vi "Calibration Helper.vi"(6 "Std Devs":cluster{"H":dbl, "S":dbl, "V":dbl}={"H"=4.0, "S"=6.0, "V"=4.0}, 7 "Image Name":string="untitled", 8 "Color Mode":u16(ring)=2 items=["RGB", "HSL", "HSV", "HSI", "CIE L*a*b*", "CIE XYZ"], 9 "Color Components":T1={"Hue"={110.0, 142.0}, "Sat"={138.0, 255.0}, "Val"={139.0, 198.0}} {"Val" scale=0.0..255.0; "Sat" scale=0.0..255.0; "Hue" scale=0.0..255.0 scale format="%#_3g"}, 10 "Image":T2, 11 "Image Ctl Refnum":refnum<vi>) -> (2 "Changed":bool, 3 "output color":T3)   [LabVIEW 2013]
uses:
  <vilib>/vision/Image Controls.llb/IMAQ Image.ctl
  <vilib>/vision/NI_Vision_Development_Module.lvlib
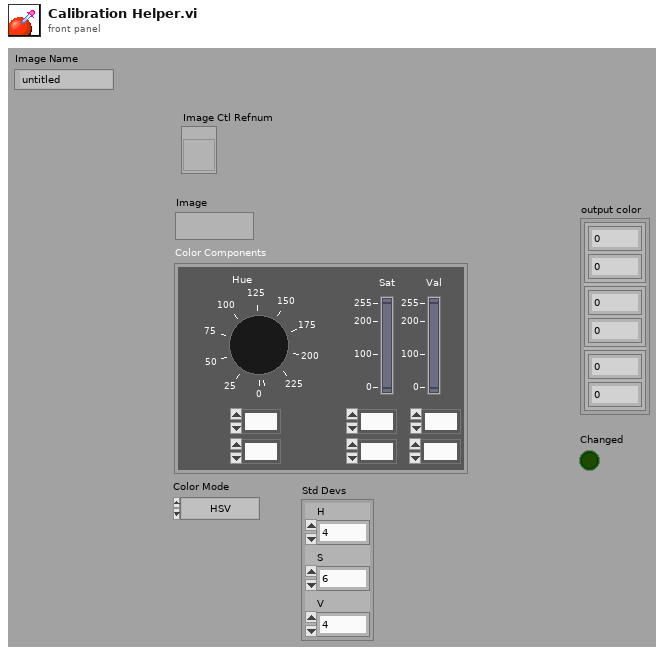
[diagram p1: front panel]
types:
  T1 = cluster{"Hue":cluster{dbl, dbl}, "Sat":cluster{dbl, dbl}, "Val":cluster{dbl, dbl}}
  T2 = typedef "IMAQ Image.ctl" = refnum<image>
  T3 = cluster{cluster{dbl, dbl}, cluster{dbl, dbl}, cluster{dbl, dbl}}
  T4 = typedef "Image Type" = u32
  T5 = cluster{"Global Rectangle":i32[], "Contours":cluster{"Contour Type":u32, "ROI Type":u32, "Points":i32[]}[]}
  T6 = cluster{"histogram":u32[], "Minimal Value":sgl, "Maximal Value":sgl, "Starting Value":sgl, "Interval Width":sgl, "Mean Value":sgl, "Standard  Variation":sgl, "Area (pixels)":i32}
  T7 = cluster{"histogram":u32[], "Minimal Value":sgl, "Maximal Value":sgl, "Starting Value":sgl, "Interval Width":sgl, "Mean Value":sgl, "Standard  Variation":sgl, "Area (pixels)":i32}[]
  T8 = cluster{"[0]":cluster{dbl, dbl}, "[1]":cluster{dbl, dbl}, "[2]":cluster{dbl, dbl}}
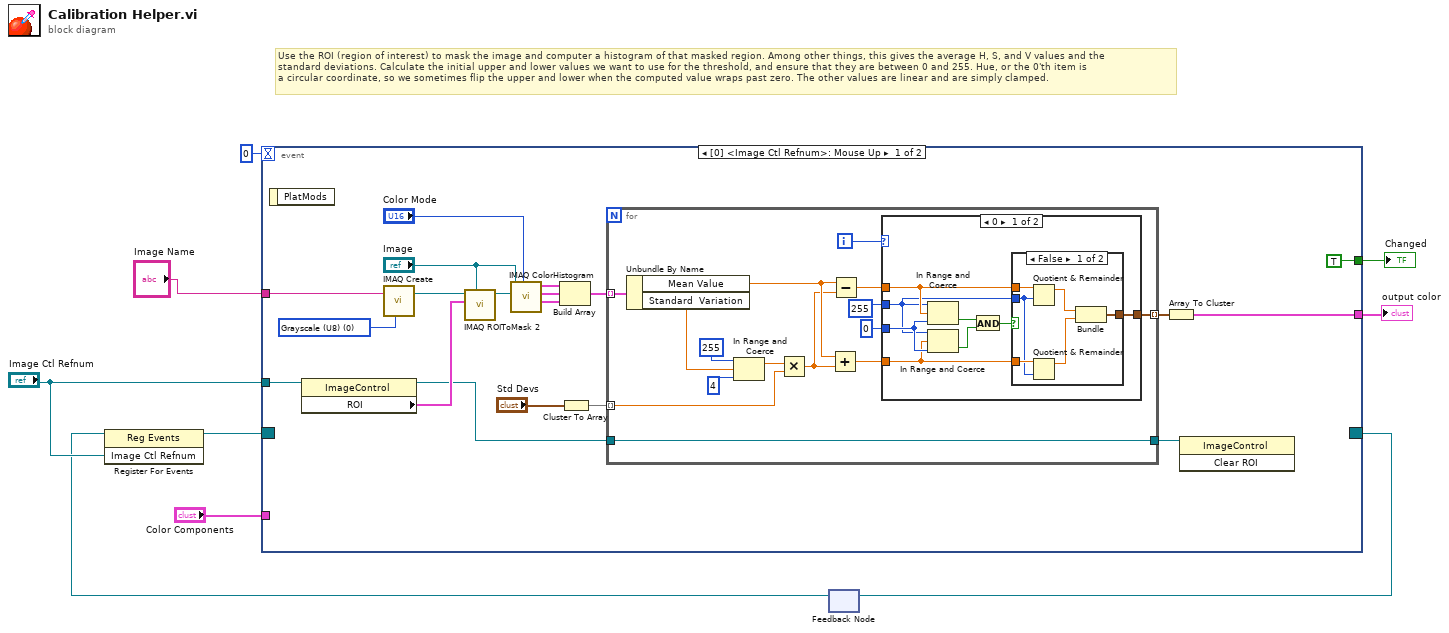
[diagram p0: block diagram]
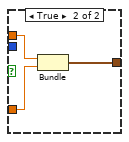
[diagram p2: hidden frame]
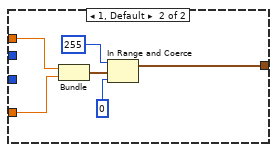
[diagram p3: hidden frame]
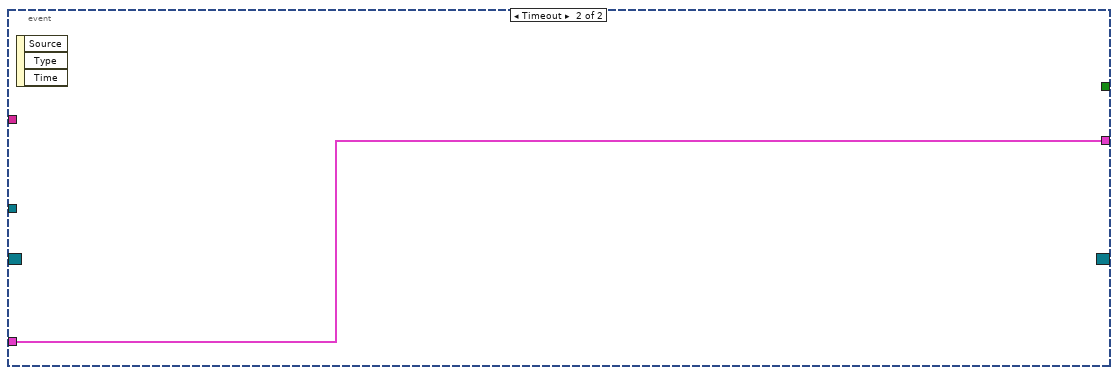
[diagram p4: hidden frame]
diagram:
  # "Use the ROI (region of interest) to mask the image and computer a histogram of that masked region. Among other things, this gives the average H, S, and V values and the\nstandard deviations. Calculate the initial upper and lower values we want to use for the threshold, and ensure that they are between 0 and 255. Hue, or the 0'th item is\na circular coordinate, so we sometimes flip the upper and lower when the computed value wraps past zero. The other values are linear and are simply clamped."
  n1 = feedback #1() -> (w3:refnum<event-registration>)  [unwired: 1 in]
  n2 = register-events(reference=w3, "Image Ctl Refnum") -> (reference out=w7:refnum<event-registration>)  [unwired: 1 in, 1 out]
  n3 = event shown="[0] <Image Ctl Refnum>: Mouse Up" {
    selector: w7 -> [_ _]
    dyn-events: [_ _] -> w4
    timeout: 0 -> [_ _]
    tunnel: "Image Ctl Refnum" -> [w16 _]
    tunnel: "Color Components" -> [_ w67]
    tunnel: [w12 w67] -> w5
    tunnel: [TRUE _] -> w2
    tunnel: "Image Name" -> [w10 _]
    event Mouse Up {
      w28 = T4 0 items=["Grayscale (U8)", "Grayscale (I16)", "Grayscale (SGL)", "Complex (CSG)", "RGB (U32)", "HSL (U32)", "RGB (U64)", "Grayscale (U16)"] ("Image Type")
      n4 = event-data() -> ()  [unwired: 1 in, 1 out]
      n5 = property on="Property Node" class="ImageControl"(reference=w16) -> (reference out=w13:refnum<vi>, "ROI"=w15:T5)  [unwired: 1 in, 1 out]
      n6 = call "IMAQ Create"("Image Name"=w10, "Image Type"=w28) -> ("New Image"=w26:T2)  [unwired: 3 in, 1 out]
      n7 = call "IMAQ ROIToMask 2"("Image Model"="Image", "ROI Descriptor"=w15, "Image"=w26) -> ("Image Out"=w27:T2)  [unwired: 6 in, 2 out]
      n8 = call "IMAQ ColorHistogram"("Color Mode"="Color Mode", "Image Src"="Image", "Image Mask"=w27) -> ("Red or Hue or X or L* Histogram Report"=w22:T6, "Green or Sat or Y or a* Histogram Report"=w21:T6, "Blue or Luma or Val or Inten or Z or b* Histogram Report"=w20:T6)  [unwired: 3 in, 1 out]
      n9 = Build Array(w22, w21, w20) -> (w18:T7)
      n10 = Cluster To Array(cluster="Std Devs") -> (array=w19:dbl[])
      n11 = for {
        tunnel: w19 -> [w39] mode=indexing
        tunnel: w18 -> [w43] mode=indexing
        tunnel: [w34] -> w17 mode=indexing
        tunnel: [w29] -> w14
        tunnel: w13 -> [w29]
        i -> [w32]
        n12 = Unbundle By Name(w43) -> ("Mean Value"=w37:sgl, "Standard  Variation"=w40:sgl)
        n13 = In Range and Coerce(upper limit=255, x=w40, lower limit=4) -> (coerced(x)=w38:sgl)  [unwired: 1 out]
        n14 = Multiply(x=w38, y=w39) -> (x*y=w33:dbl)
        n15 = Add(x=w37, y=w33) -> (x+y=w35:dbl)
        n16 = Subtract(x=w37, y=w33) -> (x-y=w36:dbl)
        n17 = case shown="0" w32 {
          tunnel: w36 -> [w46 w63]
          tunnel: w35 -> [w45 w62]
          tunnel: [w48 w61] -> w34
          tunnel: 255 -> [w44 _]
          tunnel: 0 -> [w47 _]
          frame 0 {
            n18 = In Range and Coerce(upper limit=w44, x=w46, lower limit=w47) -> (In Range?=w50:bool)  [unwired: 1 out]
            n19 = In Range and Coerce(upper limit=w44, x=w45, lower limit=w47) -> (In Range?=w49:bool)  [unwired: 1 out]
            n20 = And(x=w50, y=w49) -> (x .and. y?=w51:bool)
            n21 = case shown="False" w51 {
              tunnel: [w54 w60] -> w48
              tunnel: w46 -> [w57 w58]
              tunnel: w45 -> [w56 w59]
              tunnel: w44 -> [w55 _]
              frame False {
                n22 = Quotient & Remainder(x=w57, y=w55) -> (x-y*floor(x/y)=w52:dbl)  [unwired: 1 out]
                n23 = Quotient & Remainder(x=w56, y=w55) -> (x-y*floor(x/y)=w53:dbl)  [unwired: 1 out]
                n24 = Bundle(w52, w53) -> (w54:cluster{dbl, dbl})  [unwired: 1 in]
              }
              frame True {
                n25 = Bundle(w58, w59) -> (w60:cluster{dbl, dbl})  [unwired: 1 in]
              }
            }
          }
          frame 1, Default {
            n26 = Bundle(w63, w62) -> (w66:cluster{dbl, dbl})  [unwired: 1 in]
            n27 = In Range and Coerce(upper limit=255, x=w66, lower limit=0) -> (coerced(x)=w61:cluster{dbl, dbl})  [unwired: 1 out]
          }
        }
      }
      n28 = Array To Cluster(array=w17) -> (cluster=w12:T8)
      n29 = invoke on="Invoke Node" class="ImageControl" method="Clear ROI"(reference=w14) -> ()  [unwired: 2 in, 3 out]
    }
    event Timeout {
      n30 = event-data() -> ()  [unwired: 1 in, 3 out]
    }
  }
  "output color" <- w5
  "Changed" <- w2
  n31 = feedback-in #1(w4) -> ()
